vi "Compute Target Distances Poly.vi"   [LabVIEW 2013]
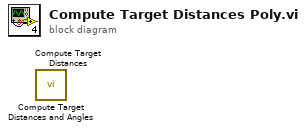
[diagram p0: block diagram]
diagram:
  n1 = call "Compute Target Distances and Angles.vi"() -> ()  [unwired: 9 in, 3 out]
  n2 = call "Compute Target Distances.vi"() -> ()  [unwired: 9 in, 3 out]
